vi "Read MinWidth.vi"(8 "error in (no error)":errorcluster, 11 "GridColumn in":refnum<class "GridColumn.lvclass">) -> (0 "error out":errorcluster, 2 "MinWidth":i32=100 min=2 step=1, 3 "GridColumn out":refnum<class "GridColumn.lvclass">)   [LabVIEW 2013, in "DataGrid.lvlib" / "GridColumn.lvclass"]
uses:
  GridColumn.lvclass
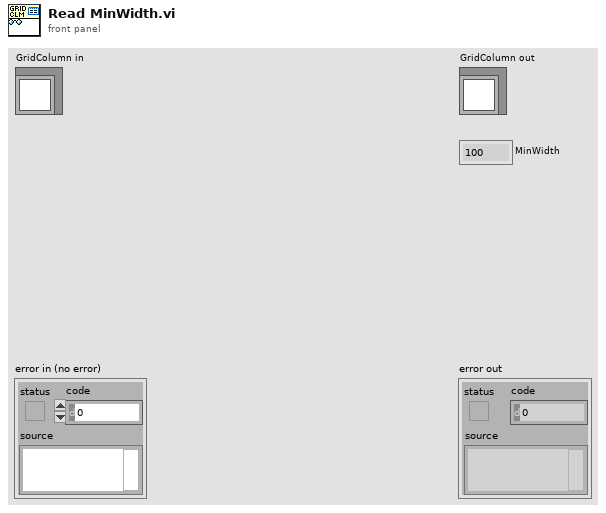
[diagram p1: front panel]
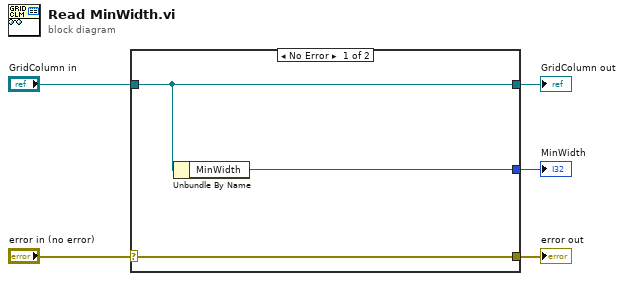
[diagram p0: block diagram]
diagram:
  n1 = case shown="No Error" "error in (no error)" {
    selector: "error in (no error)" -> [w8 w9]
    tunnel: [w8 w9] -> w4
    tunnel: [w7 w10] -> w2
    tunnel: "GridColumn in" -> [w7 w10]
    tunnel: [w6 _] -> w1
    frame No Error {
      n2 = Unbundle By Name(w7) -> ("MinWidth"=w6:i32)
    }
    frame Error {
    }
  }
  "error out" <- w4
  "GridColumn out" <- w2
  "MinWidth" <- w1
